vi "Update Library Icon.vi"(8 "error in (no error)":errorcluster, 9 "Label BG Color":u32(colorbox)=15925152, 10 "Label Text":string, 11 "Library Refnum in":refnum<vi>) -> (0 "error out":errorcluster, 3 "Library Refnum Out":refnum<vi>)   [LabVIEW 2020, in "ADAS_IO_Template_MDO.lvclass"]
uses:
  ADAS_IO_Template_MDO.lvclass
  <vilib>/LabVIEW Icon API/LabVIEW Icon API.lvlib
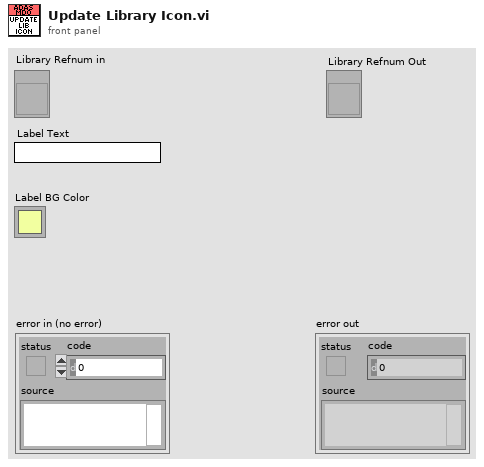
[diagram p1: front panel]
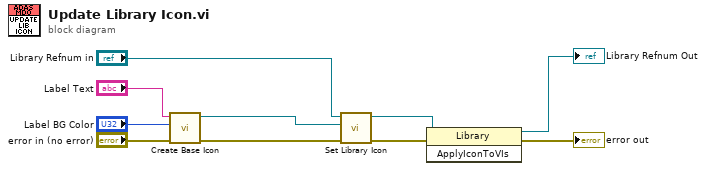
[diagram p0: block diagram]
diagram:
  n1 = call "Create Base Icon.vi"("error in (no error)"="error in (no error)", "Label BG Color"="Label BG Color", "Label Text"="Label Text") -> ("error out"=w4:errorcluster, "Icon.lvlclass out"=w3:refnum<class "Icon.lvclass">)  [unwired: 7 in]
  n2 = call <vilib>:"Set Library Icon.vi"("error in (no error)"=w4, "Icon"=w3, "Library Refnum in"="Library Refnum in") -> ("error out"=w10:errorcluster, "Library Refnum out"=w7:refnum<vi>)  [unwired: 7 in]
  n3 = invoke class="Library" method="ApplyIconToVIs"(reference=w7, error in=w10) -> (reference out=→"Library Refnum Out":refnum<vi>, error out=→"error out":errorcluster)  [unwired: 1 in, 1 out]
